vi "TemperatureHumidityMonitor.vi"() -> ()   [LabVIEW 2018]
uses:
  InstrControl/ArduinoControl/ArduinoControl.lvclass
  InstrControl/InstrumentSetup.vi
  InstrControl/InstrControl.lvclass
panel:
  in  "VISA address":refnum<visa-resource-name>="COM24"
  in  "Duration":u32=43200 step=3600 format="%<%H:%M:%S>t"
  in  "Run":bool
  in  "quit":bool
  out "Run time":u32 format="%<%H:%M:%S>t"
  out "Humidity":dbl caption="Humidity [%]"
  out "Temp.":dbl caption="Temp. [°C]"
  in  "Interval [s]":u32=10
  out "Tgraph":cluster{u32[], dbl[]}[](graph)
  # "Temperature & Humidity Monitor"
  # "University of\nCambridge"
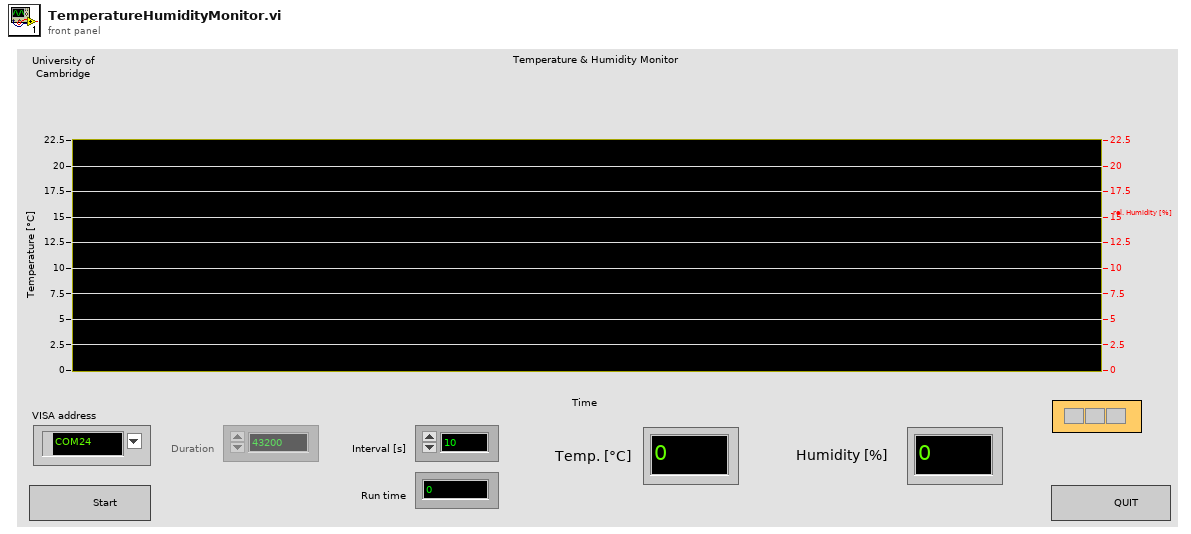
[diagram p1: front panel]
types:
  T1 = cluster{"VISA address":refnum<visa-resource-name>, "T sensor":enum16{"SHT", "DS"}, "Arduino":refnum<class "ArduinoControl.lvclass">}
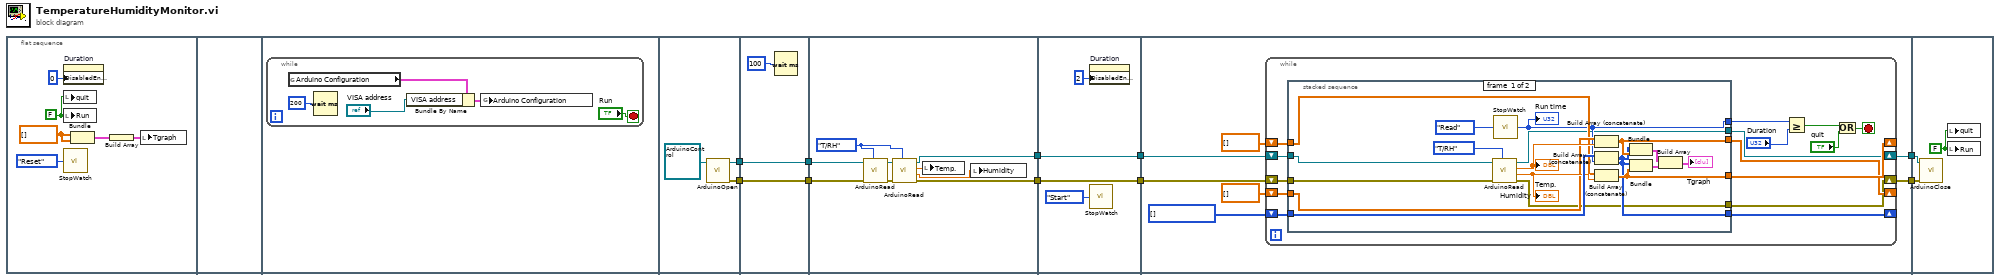
[diagram p0: block diagram]
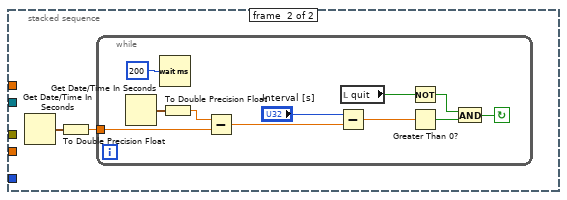
[diagram p2: hidden frame]
diagram:
  n1 = flat-sequence {
    tunnel: [w23] -> w4
    tunnel: [w22] -> w2
    tunnel: w4 -> [w27]
    tunnel: [w27] -> w3
    tunnel: w2 -> [w26]
    tunnel: [w26] -> w1
    tunnel: [w31] -> w6
    tunnel: [w30] -> w5
    tunnel: w3 -> [w29]
    tunnel: w1 -> [w28]
    tunnel: [w38] -> w10
    tunnel: [w37] -> w8
    tunnel: w6 -> [w37]
    tunnel: w5 -> [w38]
    tunnel: w10 -> [w44]
    tunnel: [w43] -> w9
    tunnel: w8 -> [w42]
    tunnel: [w41] -> w7
    tunnel: w9 -> [w95]
    tunnel: w7 -> [w94]
    frame #0 {
      w14 = dbl[] []
      w15 = FALSE
      n2 = property on="Duration" class="DigNum (strict)"("DisabledEnum"=0) -> ()  [unwired: 2 in, 2 out]
      n3 = local write "quit"(w15) -> ()
      n4 = local write "Run"(w15) -> ()
      n5 = call "StopWatch.vi"("Action"=enum16{"Start", "Stop", "Read", "Reset"}."Reset") -> ()  [unwired: 5 out]
      n6 = Bundle(w14, w14) -> (w12:cluster{dbl[], dbl[]})  [unwired: 1 in]
      n7 = Build Array(w12) -> (w13:cluster{dbl[], dbl[]}[])
      n8 = local write "Tgraph"(w13) -> ()
    }
    frame #1 {
    }
    frame #2 {
      n9 = while {
        stop <- "Run" stop-if-true
        n10 = global read "InstrumentSetup.vi" "Arduino Configuration"() -> (w17:T1)
        n11 = Wait (ms)(milliseconds to wait=u32 200) -> ()  [unwired: 1 out]
        n12 = Bundle By Name(cluster=w17, "VISA address"="VISA address") -> (w19:T1)
        n13 = global write "InstrumentSetup.vi" "Arduino Configuration"(w19) -> ()
      }
    }
    frame #3 {
      n14 = call "ArduinoOpen.vi"("ArduinoControl in"=refnum<class "ArduinoControl.lvclass"> refnum) -> ("error out"=w22:errorcluster, "ArduinoControl out"=w23:refnum<class "ArduinoControl.lvclass">)  [unwired: 9 in]
    }
    frame #4 {
      n15 = Wait (ms)(milliseconds to wait=100) -> ()  [unwired: 1 out]
    }
    frame #5 {
      w36 = enum16{"T/RH", "Interlock", "Edgesense"}."T/RH" ("Arduino function")
      n16 = call "ArduinoRead.vi"("Arduino function"=w36, "error in (no error)"=w28, "ArduinoControl in"=w29) -> ("error out"=w35:errorcluster, "ArduinoControl out"=w34:refnum<class "ArduinoControl.lvclass">)  [unwired: 3 in, 4 out]
      n17 = call "ArduinoRead.vi"("Arduino function"=w36, "error in (no error)"=w35, "ArduinoControl in"=w34) -> ("error out"=w31:errorcluster, "rel. Humidity [%]"=w32:dbl, "Temperature [°C]"=w33:dbl, "ArduinoControl out"=w30:refnum<class "ArduinoControl.lvclass">)  [unwired: 3 in, 2 out]
      n18 = local write "Temp."(w33) -> ()
      n19 = local write "Humidity"(w32) -> ()
    }
    frame #6 {
      n20 = property on="Duration" class="DigNum (strict)"("DisabledEnum"=2) -> ()  [unwired: 2 in, 2 out]
      n21 = call "StopWatch.vi"("Action"=enum16{"Start", "Stop", "Read", "Reset"}."Start") -> ()  [unwired: 5 out]
    }
    frame #7 {
      n22 = while {
        shift-right: [w57] -> _
        shift-left: u32[] [] -> [w58]
        shift-right: [w53] -> _
        shift-left: dbl[] [] -> [w56]
        shift-right: [w54] -> _
        shift-left: dbl[] [] -> [w55]
        shift-right: [w50] -> w43
        shift-left: w44 -> [w51]
        shift-right: [w48] -> w41
        shift-left: w42 -> [w49]
        stop <- w59 stop-if-true
        n23 = stacked-sequence {
          tunnel: w58 -> [w79 _]
          tunnel: [w72 _] -> w57
          tunnel: w56 -> [w76 _]
          tunnel: w55 -> [w75 _]
          tunnel: [w74 _] -> w54
          tunnel: [w73 _] -> w53
          tunnel: [w68 _] -> w52
          tunnel: w51 -> [w67 _]
          tunnel: [w66 _] -> w50
          tunnel: w49 -> [w65 _]
          tunnel: [w64 _] -> w48
          frame #0 {
            n24 = call "ArduinoRead.vi"("Arduino function"=enum16{"T/RH", "Interlock", "Edgesense"}."T/RH", "error in (no error)"=w65, "ArduinoControl in"=w67) -> ("error out"=w64:errorcluster, "rel. Humidity [%]"=w78:dbl, "Temperature [°C]"=w77:dbl, "ArduinoControl out"=w66:refnum<class "ArduinoControl.lvclass">)  [unwired: 3 in, 2 out]
            "Humidity" <- w78
            "Temp." <- w77
            n25 = call "StopWatch.vi"("Action"=enum16{"Start", "Stop", "Read", "Reset"}."Read") -> ("Time elapsed"=w68:u32)  [unwired: 4 out]
            "Run time" <- w68
            n26 = Build Array (concatenate)(w76, w77) -> (w73:dbl[])
            n27 = Build Array (concatenate)(w79, w68) -> (w72:u32[])
            n28 = Build Array (concatenate)(w75, w78) -> (w74:dbl[])
            n29 = Bundle(w72, w73) -> (w71:cluster{u32[], dbl[]})  [unwired: 1 in]
            n30 = Bundle(w72, w74) -> (w70:cluster{u32[], dbl[]})  [unwired: 1 in]
            n31 = Build Array(w71, w70) -> (→"Tgraph":cluster{u32[], dbl[]}[])
          }
          frame #1 {
            n32 = Get Date/Time In Seconds() -> (seconds since 1Jan1904=w82:timestamp)
            n33 = To Double Precision Float(number=w82) -> (double precision float=w81:dbl)
            n34 = while {
              tunnel: w81 -> [w90]
              stop <- w83 continue-if-true
              n35 = Get Date/Time In Seconds() -> (seconds since 1Jan1904=w92:timestamp)
              n36 = Wait (ms)(milliseconds to wait=u32 200) -> ()  [unwired: 1 out]
              n37 = To Double Precision Float(number=w92) -> (double precision float=w91:dbl)
              n38 = Subtract(x=w91, y=w90) -> (x-y=w89:dbl)
              n39 = Subtract(x="Interval [s]", y=w89) -> (x-y=w87:dbl)
              n40 = local read "quit"() -> (w86:bool)
              n41 = Not(x=w86) -> (.not. x?=w85:bool)
              n42 = Greater Than 0?(x=w87) -> (x > 0?=w84:bool)
              n43 = And(x=w85, y=w84) -> (x .and. y?=w83:bool)
            }
          }
        }
        n44 = Greater Or Equal?(x=w52, y="Duration") -> (x >= y?=w60:bool)
        n45 = Or(x=w60, y="quit") -> (x .or. y?=w59:bool)
      }
    }
    frame #8 {
      w96 = FALSE
      n46 = call "ArduinoClose.vi"("error in (no error)"=w94, "ArduinoControl in"=w95) -> ()  [unwired: 8 in, 2 out]
      n47 = local write "quit"(w96) -> ()
      n48 = local write "Run"(w96) -> ()
    }
  }
